vi "Launch Helm Actor.vi"(11 "RDS Root Actor in":refnum<class "RDS Root Actor.lvclass">) -> (3 "RDS Root Actor out":refnum<class "RDS Root Actor.lvclass">)   [LabVIEW 2015, in "RDS Root Actor.lvlib" / "RDS Root Actor.lvclass"]
uses:
  RDS Root Actor.lvclass
  RDS Helm Actor/RDS Helm Actor/RDS Helm Actor.lvclass
  Libraries/RDS Framework/RDS Message ID.ctl
  RDS Helm Actor/RDS Helm Actor/RDS Helm Actor.lvclass/RDS Helm Actor.ctl
  RDS Parent Actor/RDS Parent Actor/RDS Parent Actor.lvclass/RDS Parent Actor.ctl
  RDS Parent Actor/RDS Parent Actor/RDS Parent Actor.lvclass
  Libraries/Configuration Library/RDS Configuration Library.lvlib
  Libraries/RDS Child Messages/RDS Child Messages.lvlib
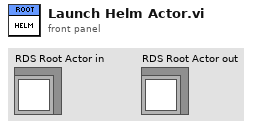
[diagram p1: front panel]
types:
  T1 = typedef "RDS Child Messages.lvlib/RDS Message ID.ctl" = enum16{"RDS Hello World", "String Message", "AIP_Status", "AIP_Command", "GPS_Data", "MCB_Command", "MCB_Status", "Compass_Data", "Depth_Data", "Battery_Data", "Contoller_State", "Set_Mag_Dev", "BTB_Shutdown", "State_Sample_Request", "State_Sample", "PID_Gains_Set", "Helm_Limiter_Set", "Helm_Heading_Command", "Helm_Steering_Command", "Helm_Status", "Controller_Message", "AIP_Set_Min_Depth", "Mission_Controller_State", "Mission_Upload", "Mission_Set_Op_and_Run", "Mission_Settings_Set"}
  T2 = typedef "RDS Configuration Library.lvlib/RDS Configuration.ctl" = cluster{"State Update Rate (Hz)":dbl, "Helm Rate (Hz)":dbl, "Helm Gains":T3, "Limiter":dbl, "Mission Controller Settings":T4, "Mag Dev":dbl}
  T3 = typedef "RDS Child Messages.lvlib/PID Gains Control.ctl" = cluster{"P (Kc)":sgl, "I (Ti)":sgl, "D (Td)":sgl}
  T4 = typedef "RDS Mission Controller Actor.lvlib/Mission Controller Settings.ctl" = cluster{"Waypoint Radius (m)":dbl}
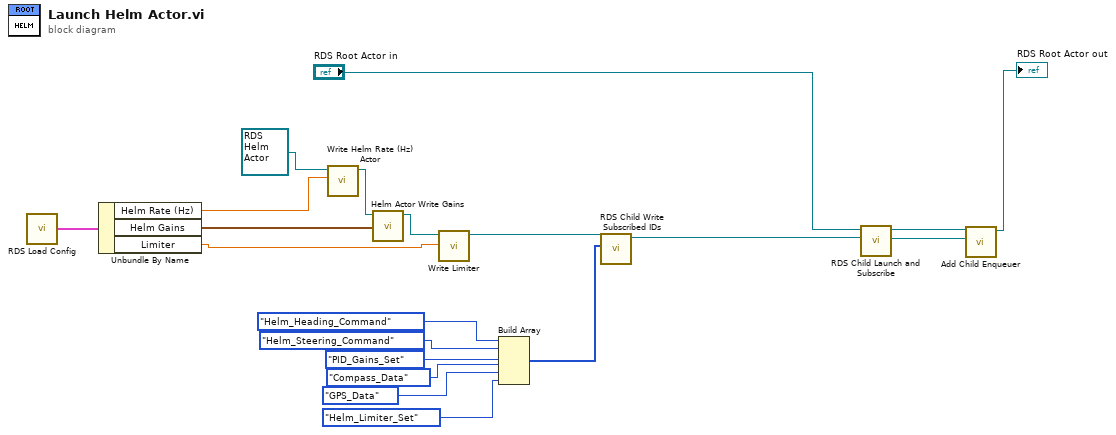
[diagram p0: block diagram]
diagram:
  n1 = call "RDS Load Config.vi"() -> ("RDS Config"=w15:T2)  [unwired: 11 in]
  n2 = Unbundle By Name(w15) -> ("Helm Rate (Hz)"=w11:dbl, "Helm Gains"=w12:T3, "Limiter"=w2:dbl)
  n3 = call "Write Helm Rate (Hz) Actor.vi"("Helm Rate (Hz)"=w11, "RDS Helm Actor in"=refnum<class "RDS Helm Actor.lvclass"> refnum ("RDS Helm Actor.lvlib:RDS Helm Actor.lvclass")) -> ("RDS Helm Actor out"=w13:refnum<class "RDS Helm Actor.lvclass">)  [unwired: 8 in, 1 out]
  n4 = call "Helm Actor Write Gains.vi"("Gains"=w12, "RDS Helm Actor in"=w13) -> ("RDS Helm Actor out"=w4:refnum<class "RDS Helm Actor.lvclass">)  [unwired: 8 in, 1 out]
  n5 = call "Write Limiter.vi"("Limiter"=w2, "RDS Helm Actor in"=w4) -> ("RDS Helm Actor out"=w3:refnum<class "RDS Helm Actor.lvclass">)  [unwired: 8 in, 1 out]
  n6 = Build Array(RDS_Message_ID."Helm_Heading_Command" ("RDS Message"), RDS_Message_ID."Helm_Steering_Command" ("RDS Message"), RDS_Message_ID."PID_Gains_Set" ("RDS Message"), RDS_Message_ID."Compass_Data" ("RDS Message"), RDS_Message_ID."GPS_Data" ("RDS Message"), RDS_Message_ID."Helm_Limiter_Set" ("RDS Message")) -> (w7:T1[])
  n7 = call "RDS Child Write Subscribed IDs.vi"("Subscribed IDs"=w7, "RDS Parent Actor in"=w3) -> ("RDS Parent Actor out"=w17:refnum<class "RDS Helm Actor.lvclass">)  [unwired: 8 in, 1 out]
  n8 = call "RDS Child Launch and Subscribe.vi"("RDS Child in"=w17, "Caller Actor in"="RDS Root Actor in") -> ("Nested Actor's Enqueuer"=w19:refnum<class "Message Enqueuer.lvclass">, "Caller Actor Out"=w18:refnum<class "RDS Root Actor.lvclass">)  [unwired: 7 in, 1 out]
  n9 = call "Add Child Enqueuer.vi"("Nested Actor's Enqueuer"=w19, "RDS Root Actor in"=w18) -> ("RDS Root Actor out"=→"RDS Root Actor out":refnum<class "RDS Root Actor.lvclass">)  [unwired: 8 in, 1 out]
